vi "Post-Build Action.vi"(5 "Files Generated by Build":path[](array[path]), 6 "Top Level/Always Included VIs":path[](array[path]), 7 "Destination Path":path, 8 "error in (no error)":errorcluster, 9 "Target Name":string, 10 "Build Specification Name":string, 11 "Project Path":path) -> (0 "error out":errorcluster)   [LabVIEW 2018]
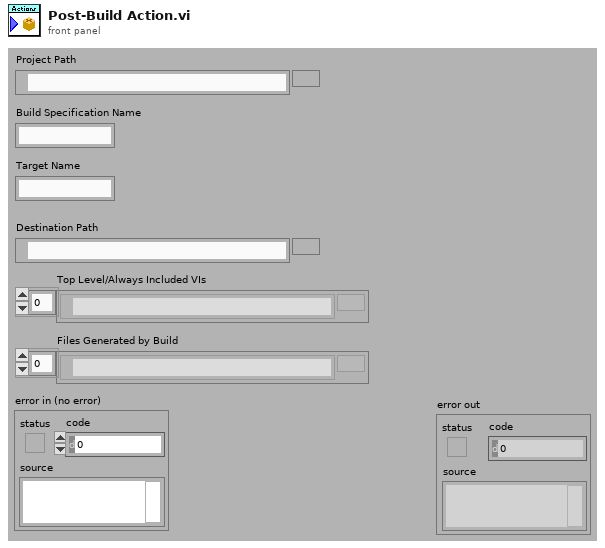
[diagram p1: front panel]
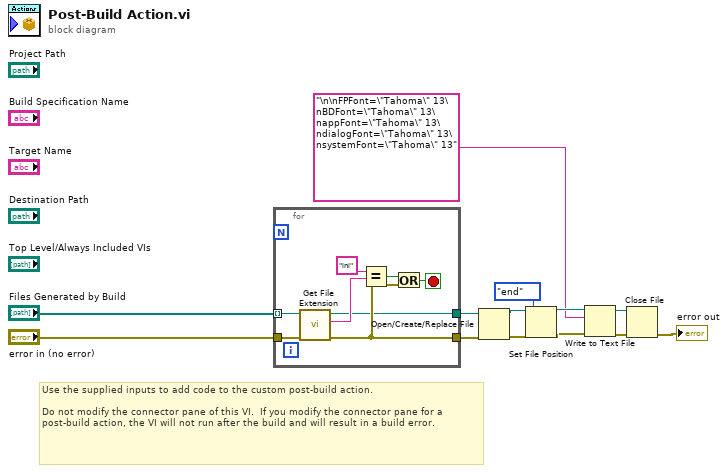
[diagram p0: block diagram]
diagram:
  # "Use the supplied inputs to add code to the custom post-build action.\n\nDo not modify the connector pane of this VI.  If you modify the connector pane for a post-build action, the VI will not run after the build and will result in a build error."
  n1 = for {
    tunnel: "Files Generated by Build" -> [w21] mode=indexing
    tunnel: [w15] -> w4
    tunnel: "error in (no error)" -> [w17]
    tunnel: [w14] -> w1
    stop <- w16 stop-if-true
    n2 = call <vilib>:"Get File Extension.vi"("error in (no error)"=w17, "file"=w21) -> ("error out"=w15:errorcluster, "lowercase file extension"=w20:string, "dup file"=w14:path)  [unwired: 5 in, 2 out]
    n3 = Equal?(x="ini" ("y"), y=w20) -> (x = y?=w18:bool)
    n4 = Or(x=w18, y=w15) -> (x .or. y?=w16:bool)
  }
  n5 = Open/Create/Replace File(file path (use dialog)=w1, error in=w4) -> (refnum out=w12:refnum<file>, error out=w10:errorcluster)  [unwired: 4 in, 1 out]
  n6 = Set File Position(refnum=w12, from (0:start)=enum16{"start", "end", "current"}."end", error in=w10) -> (refnum out=w6:refnum<file>, error out=w9:errorcluster)  [unwired: 1 in]
  n7 = Write to Text File(file (use dialog)=w6, text="\n\nFPFont=\"Tahoma\" 13\nBDFont=\"Tahoma\" 13\nappFont=\"Tahoma\" 13\ndialogFont=\"Tahoma\" 13\nsystemFont=\"Tahoma\" 13", error in=w9) -> (refnum out=w7:refnum<file>, error out=w8:errorcluster)  [unwired: 1 in, 1 out]
  n8 = Close File(refnum=w7, error in=w8) -> (error out=→"error out":errorcluster)  [unwired: 1 out]
